vi "UserDefinedQNames.vi"() -> (2 "All Queues":T1)   [LabVIEW 2016]
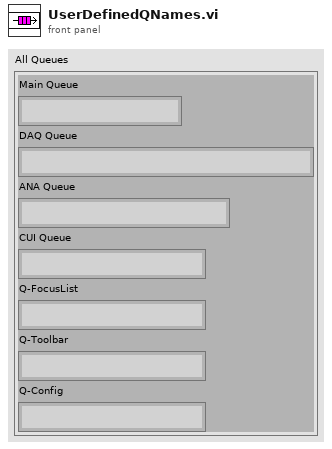
[diagram p1: front panel]
types:
  T1 = cluster{"Main Queue":string, "DAQ Queue":string, "ANA Queue":string, "CUI Queue":string, "Q-FocusList":string, "Q-Toolbar":string, "Q-Config":string}
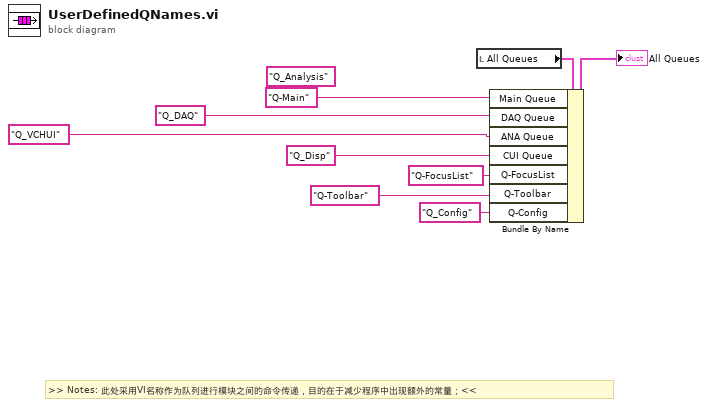
[diagram p0: block diagram]
diagram:
  (unwired) "Q_Analysis" ("Queue name(unamed)")
  # ">> Notes: 此处采用VI名称作为队列进行模块之间的命令传递，目的在于减少程序中出现额外的常量；<<"
  n1 = local read "All Queues"() -> (w5:T1)
  n2 = Bundle By Name(cluster=w5, "Main Queue"="Q-Main", "DAQ Queue"="Q_DAQ" ("Name"), "ANA Queue"="Q_VCHUI" ("Name"), "CUI Queue"="Q_Disp" ("QueueName"), "Q-FocusList"="Q-FocusList", "Q-Toolbar"="Q-Toolbar", "Q-Config"="Q_Config") -> (→"All Queues":T1)
